vi "Z factor.vi"(6 "BP":dbl[](array[numeric]), 9 "BN":dbl[](array[numeric]), 10 "AN":dbl[](array[numeric]), 11 "Parameters":T1 {"Delta 1" step=0.001 format="%#_6peV"; "Resolution" format="%#_6peV"; "Integration range" format="%#_6peV"; "T" format="%#_6pK"; "Delta 2" step=0.001 format="%#_6peV"; "Gama" step=0.001 format="%#_6peV"}) -> (2 "z factor":dbl[](array[numeric]))   [LabVIEW 2021]
uses:
  Parameters.ctl
panel:
  in  "dV":dbl
  out "Waveform Graph":cluster{dbl, "dV":dbl, dbl[][]}(graph)
  # "<="
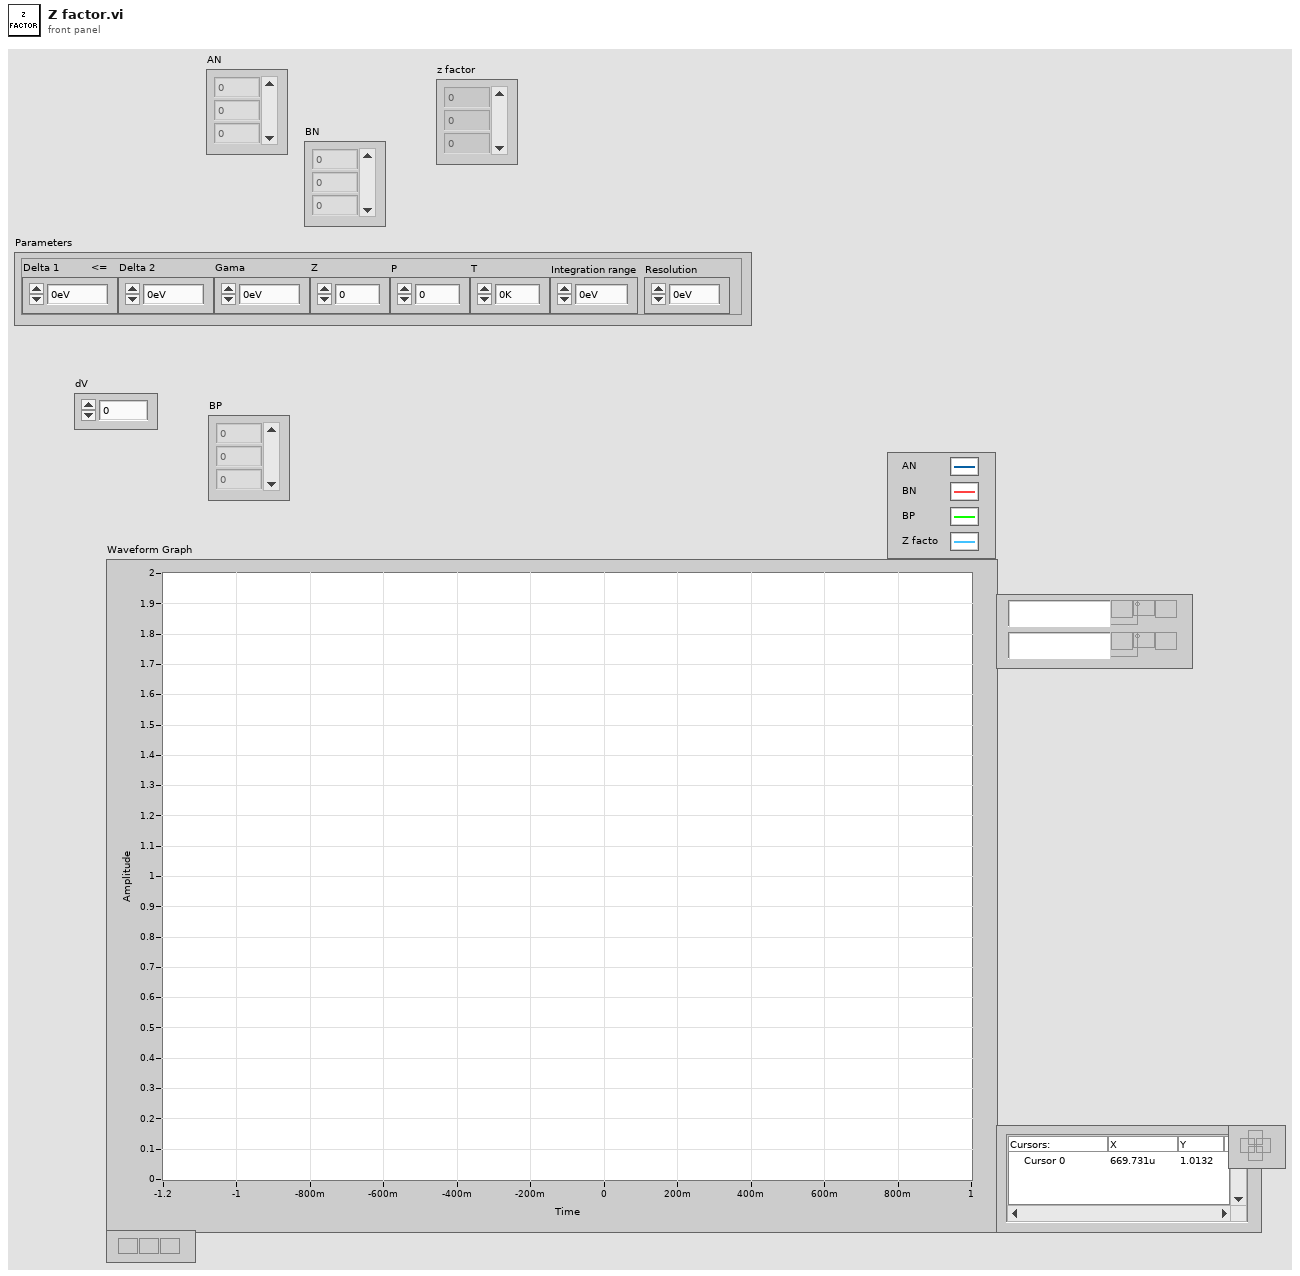
[diagram p1: front panel]
types:
  T1 = typedef "Parameters.ctl" = cluster{"Delta 1":dbl, "Delta 2":dbl, "Gama":dbl, "Z":dbl, "P":dbl, "T":dbl, "Integration range":dbl, "Resolution":dbl}
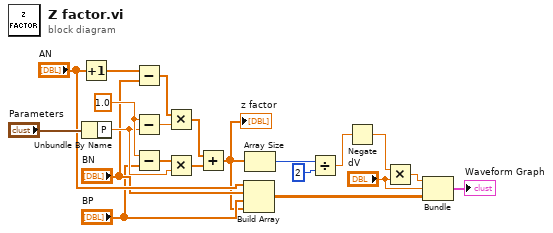
[diagram p0: block diagram]
diagram:
  w17 = 1.0 ("x")
  n1 = Increment(x="AN") -> (x+1=w20:dbl[])
  n2 = Unbundle By Name("Parameters") -> ("P"=w15:dbl)
  n3 = Subtract(x=w20, y="BN") -> (x-y=w19:dbl[])
  n4 = Subtract(x=w17, y=w15) -> (x-y=w18:dbl)
  n5 = Subtract(x=w17, y="BP") -> (x-y=w16:dbl[])
  n6 = Multiply(x=w19, y=w18) -> (x*y=w14:dbl[])
  n7 = Multiply(x=w16, y=w15) -> (x*y=w13:dbl[])
  n8 = Add(x=w14, y=w13) -> (x+y=w7:dbl[])
  "z factor" <- w7
  n9 = Build Array("AN", "BN", "BP", w7) -> (w9:dbl[][])
  n10 = Array Size(array=w7) -> (size(s)=w6:i32)
  n11 = Divide(x=w6, y=2) -> (x/y=w4:dbl)
  n12 = Negate(x=w4) -> (-x=w3:dbl)
  n13 = Multiply(x=w3, y="dV") -> (x*y=w2:dbl)
  n14 = Bundle(w2, "dV"="dV", w9) -> (→"Waveform Graph":cluster{dbl, "dV":dbl, dbl[][]})  [unwired: 1 in]
